vi "Error Handler.vi"(7 "Log?":bool=TRUE, 11 "error in (no error)":errorcluster) -> (8 "error?":bool, 10 "Details":string, 15 "No Error":errorcluster)   [LabVIEW 2020]
uses:
  Error-Library Action.ctl
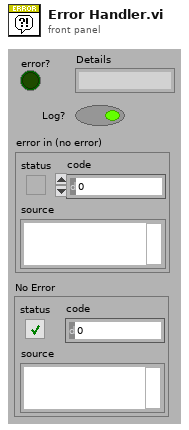
[diagram p1: front panel]
types:
  T1 = typedef "Error-Library Action.ctl" = enum16{"NONE", "Register", "Read"}
  T2 = typedef "Error Description.ctl" = cluster{"Code":i32, "Description":string, "Details":string}
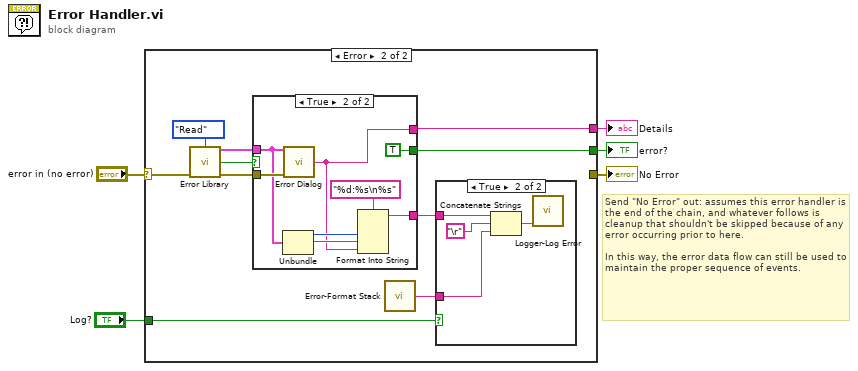
[diagram p0: block diagram]
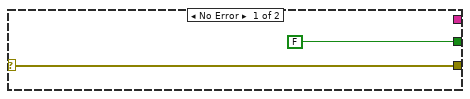
[diagram p2: hidden frame]
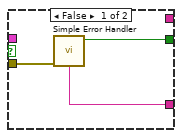
[diagram p3: hidden frame]
diagram:
  # "Send \"No Error\" out: assumes this error handler is the end of the chain, and whatever follows is cleanup that shouldn't be skipped because of any error occurring prior to here.\n\nIn this way, the error data flow can still be used to maintain the proper sequence of events."
  n1 = case shown="Error" "error in (no error)" {
    selector: "error in (no error)" -> [w6 w16]
    tunnel: [FALSE ("error?") w17] -> w4
    tunnel: [w6 _] -> w3
    tunnel: [_ w11] -> w2
    tunnel: "Log?" -> [_ w10]
    frame No Error {
    }
    frame Error {
      n2 = call "Error Library.vi"("action"=Error-Library_Action."Read", "error in"=w16) -> ("Entry"=w14:T2, "found?"=w12:bool, "error thru"=w13:errorcluster)  [unwired: 11 in]
      n3 = case shown="True" w12 {
        tunnel: w13 -> [w20 w28]
        tunnel: [w19 TRUE ("error?")] -> w17
        tunnel: w14 -> [_ w26]
        tunnel: [_ w21] -> w11
        tunnel: [w18 w23] -> w9
        frame False {
          n4 = call <vilib>:"Simple Error Handler.vi"("error in (no error)"=w20) -> ("error?"=w19:bool, "message"=w18:string)  [unwired: 4 in, 3 out]
        }
        frame True {
          n5 = Unbundle(w26) -> ("Code"=w25:i32, "Description"=w24:string)  [unwired: 1 out]
          n6 = call "Error Dialog.vi"("error"=w26, "error in (no error)"=w28) -> ("Details"=w21:string)  [unwired: 13 in]
          n7 = Format Into String(format string="%d:%s\n%s", w25, w24, w21) -> (resulting string=w23:string)  [unwired: 2 in, 1 out]
        }
      }
      n8 = call "Error-Format Stack.vi"() -> ("formatted stack"=w8:string)  [unwired: 15 in]
      n9 = case shown="True" w10 {
        tunnel: w9 -> [_ w32]
        tunnel: w8 -> [_ w30]
        frame False {
        }
        frame True {
          n10 = Concatenate Strings(w32, "\r", w30) -> (w29:string)
          n11 = call "Logger-Log Error.vi"("Message"=w29) -> ()  [unwired: 14 in, 1 out]
        }
      }
    }
  }
  "error?" <- w4
  "No Error" <- w3
  "Details" <- w2
